vi "p1.vi"() -> ()   [LabVIEW 2023, in "d24.lvlib"]
uses:
  d24.lvlib
  AOC/AOC.lvlib
panel:
  in  "Example":string="19, 13, 30 @ -2,  1, -2\n18, 19, 22 @ -1, -1, -2\n20, 25, 34 @ -2, -2, -4\n12, 31, 28 @ -1, -2, -1\n20, 19, 15 @  1, -5, -3"
  in  "Example":bool=TRUE
  out "Answer":i64=10
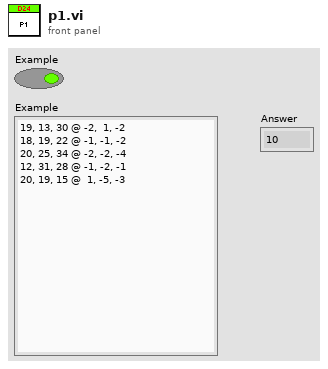
[diagram p1: front panel]
types:
  T1 = cluster{"default value 1":i64, "default value 1":i64, i64, i64, dbl, dbl}
  T2 = cluster{"default value 1":i64, "default value 1":i64}
  T3 = cluster{"default value 1":i64, "default value 1":i64, i64, i64, dbl, dbl}[]
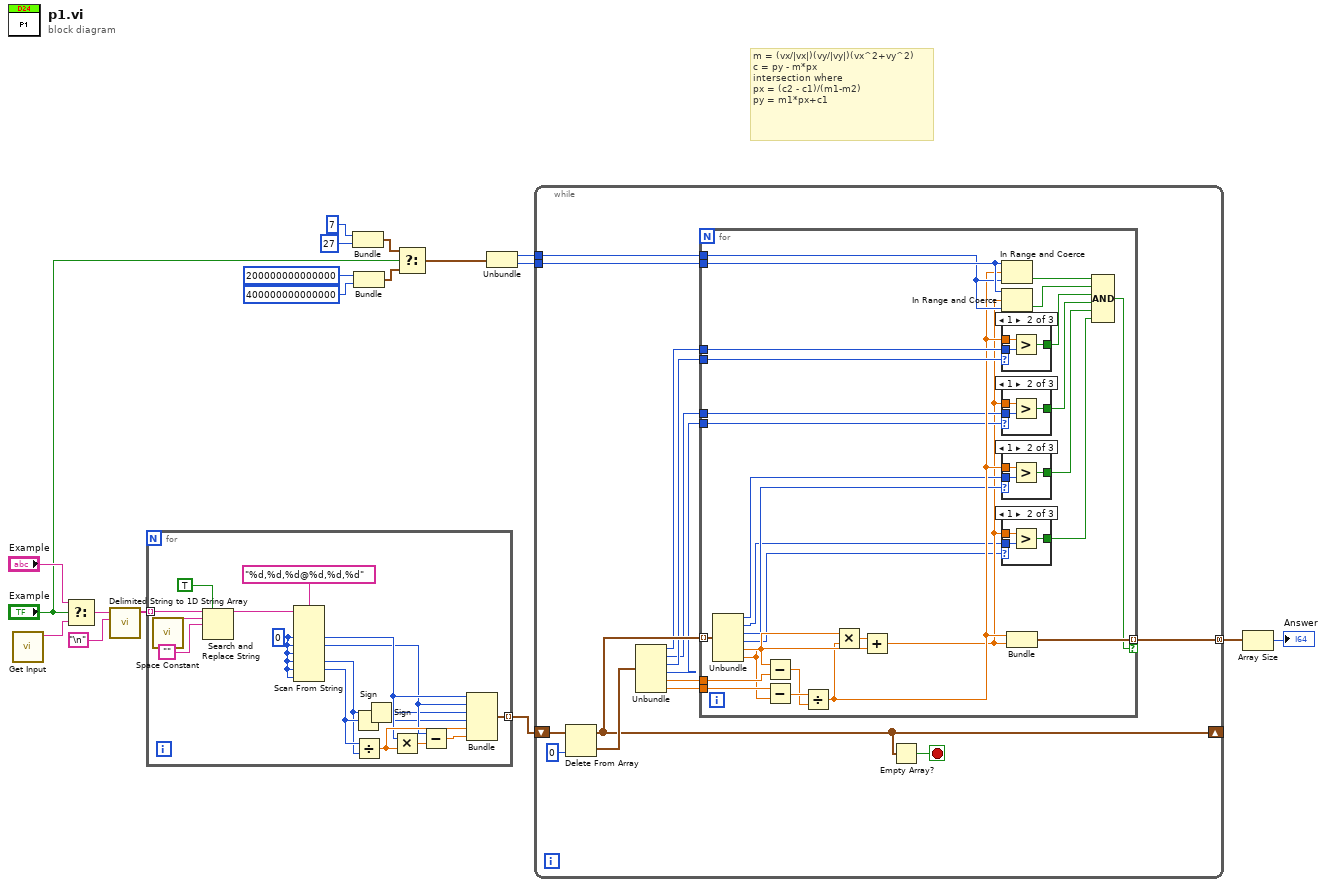
[diagram p0: block diagram]
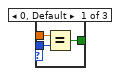
[diagram p2: hidden frame]
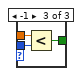
[diagram p3: hidden frame]
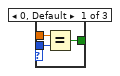
[diagram p4: hidden frame]
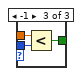
[diagram p5: hidden frame]
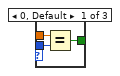
[diagram p6: hidden frame]
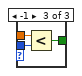
[diagram p7: hidden frame]
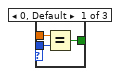
[diagram p8: hidden frame]
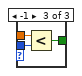
[diagram p9: hidden frame]
diagram:
  # "m = (vx/|vx|)(vy/|vy|)(vx^2+vy^2)\nc = py - m*px\nintersection where\npx = (c2 - c1)/(m1-m2)\npy = m1*px+c1"
  n1 = call "Get Input.vi"() -> ("Input"=w18:string)  [unwired: 11 in]
  n2 = Select(t="Example", s="Example", f=w18) -> (s? t:f=w16:string)
  n3 = call <vilib>:"Delimited String to 1D String Array.vi"("delimiter"="\n", "delimited string"=w16) -> ("string array"=w14:string[])  [unwired: 9 in]
  n4 = for {
    tunnel: w14 -> [w33] mode=indexing
    tunnel: [w28] -> w6 mode=indexing
    w29 = i64 0 ("default value 1")
    n5 = call <vilib>:"Space Constant.vi"() -> ("String"=w32:string)
    n6 = Search and Replace String(replace all?=TRUE ("replace all? (F)"), input string=w33, search string=w32, replace string="") -> (result string=w34:string)  [unwired: 4 in, 3 out]
    n7 = Scan From String(format string="%d,%d,%d@%d,%d,%d", input string=w34, default 1=w29, default 2=w29, default 3=w29, default 4=w29, default 5=w29, default 6=w29) -> (output 1=w24:i64, output 2=w23:i64, output 4=w21:i64, output 5=w22:i64)  [unwired: 4 in, 3 out]
    n8 = Sign(1:w22) -> (0:w19:i64)
    n9 = Divide(x=w22, y=w21) -> (x/y=w25:dbl)
    n10 = Sign(1:w21) -> (0:w20:i64)
    n11 = Multiply(x=w24, y=w25) -> (x*y=w27:dbl)
    n12 = Subtract(x=w23, y=w27) -> (x-y=w26:dbl)
    n13 = Bundle("default value 1"=w24, "default value 1"=w23, w20, w19, w25, w26) -> (w28:T1)  [unwired: 1 in]
  }
  n14 = Bundle("default value 1"=i64 7, "default value 1"=i64 27) -> (w11:T2)  [unwired: 1 in]
  n15 = Bundle("default value 1"=i64 200000000000000, "default value 1"=i64 400000000000000) -> (w7:T2)  [unwired: 1 in]
  n16 = Select(t=w11, s="Example", f=w7) -> (s? t:f=w5:T2)
  n17 = Unbundle(w5) -> ("default value 1"=w4:i64, "default value 1"=w3:i64)
  n18 = while {
    shift-right: [w45] -> _
    shift-left: w6 -> [w49]
    tunnel: w4 -> [w47]
    tunnel: w3 -> [w46]
    tunnel: [w43] -> w2 mode=concatenating
    stop <- w44 stop-if-true
    n19 = Delete From Array(array=w49, index=0) -> (deleted portion=w48:T1, array with subset deleted=w45:T3)  [unwired: 1 in]
    n20 = Unbundle(w48) -> ("default value 1"=w38:i64, "default value 1"=w37:i64, w39:i64, w36:i64, w41:dbl, w40:dbl)
    n21 = for {
      tunnel: w45 -> [w77] mode=indexing
      tunnel: w40 -> [w75]
      tunnel: w41 -> [w74]
      tunnel: w47 -> [w67]
      tunnel: w46 -> [w68]
      tunnel: [w71] -> w43 mode=indexing if=w50
      tunnel: w39 -> [w64]
      tunnel: w38 -> [w63]
      tunnel: w37 -> [w59]
      tunnel: w36 -> [w58]
      n22 = Unbundle(w77) -> ("default value 1"=w61:i64, "default value 1"=w56:i64, w60:i64, w55:i64, w66:dbl, w65:dbl)
      n23 = Subtract(x=w66, y=w74) -> (x-y=w73:dbl)
      n24 = Subtract(x=w75, y=w65) -> (x-y=w76:dbl)
      n25 = Divide(x=w76, y=w73) -> (x/y=w62:dbl)
      n26 = Multiply(x=w66, y=w62) -> (x*y=w72:dbl)
      n27 = Add(x=w72, y=w65) -> (x+y=w57:dbl)
      n28 = In Range and Coerce(upper limit=w68, x=w62, lower limit=w67) -> (In Range?=w69:bool)  [unwired: 1 out]
      n29 = In Range and Coerce(upper limit=w68, x=w57, lower limit=w67) -> (In Range?=w70:bool)  [unwired: 1 out]
      n30 = case shown="1" w64 {
        tunnel: w62 -> [w106 w110 w113]
        tunnel: w63 -> [w107 w109 w112]
        tunnel: [w105 w108 w111] -> w54
        frame 0, Default {
          n31 = Equal?(x=w106, y=w107) -> (x = y?=w105:bool)
        }
        frame 1 {
          n32 = Greater?(x=w110, y=w109) -> (0:w108:bool)
        }
        frame -1 {
          n33 = Less?(x=w113, y=w112) -> (x < y?=w111:bool)
        }
      }
      n34 = case shown="1" w58 {
        tunnel: w57 -> [w88 w92 w95]
        tunnel: w59 -> [w89 w91 w94]
        tunnel: [w87 w90 w93] -> w53
        frame 0, Default {
          n35 = Equal?(x=w88, y=w89) -> (x = y?=w87:bool)
        }
        frame 1 {
          n36 = Greater?(x=w92, y=w91) -> (0:w90:bool)
        }
        frame -1 {
          n37 = Less?(x=w95, y=w94) -> (x < y?=w93:bool)
        }
      }
      n38 = case shown="1" w60 {
        tunnel: w62 -> [w97 w101 w104]
        tunnel: w61 -> [w98 w100 w103]
        tunnel: [w96 w99 w102] -> w52
        frame 0, Default {
          n39 = Equal?(x=w97, y=w98) -> (x = y?=w96:bool)
        }
        frame 1 {
          n40 = Greater?(x=w101, y=w100) -> (0:w99:bool)
        }
        frame -1 {
          n41 = Less?(x=w104, y=w103) -> (x < y?=w102:bool)
        }
      }
      n42 = case shown="1" w55 {
        tunnel: w57 -> [w79 w83 w86]
        tunnel: w56 -> [w80 w82 w85]
        tunnel: [w78 w81 w84] -> w51
        frame 0, Default {
          n43 = Equal?(x=w79, y=w80) -> (x = y?=w78:bool)
        }
        frame 1 {
          n44 = Greater?(x=w83, y=w82) -> (0:w81:bool)
        }
        frame -1 {
          n45 = Less?(x=w86, y=w85) -> (x < y?=w84:bool)
        }
      }
      n46 = Bundle(w62, w57) -> (w71:cluster{dbl, dbl})  [unwired: 1 in]
      n47 = Compound Arithmetic op=AND(w69, w70, w54, w53, w52, w51) -> (w50:bool)
    }
    n48 = Empty Array?(array=w45) -> (empty?=w44:bool)
  }
  n49 = Array Size(array=w2) -> (size(s)=→"Answer":i32)
